vi "GE 5565PIORC.PIO.Endianness.vi"(11 "data type":T1=enum."Single") -> (0 "error out":errorcluster, 3 "pass?":bool)   [LabVIEW 2017]
uses:
  Typedefs/GE 5565PIORC.Data Types.ctl
  Source/GE 5565PIORC.lvclass/GE 5565PIORC.ctl
  Source/Methods/GE 5565PIORC.PIO.Write (SGL).vi
  Source/Methods/GE 5565PIORC.PIO.Read (SGL).vi
  Source/Methods/GE 5565PIORC.PIO.Write (DBL).vi
  Source/Methods/GE 5565PIORC.PIO.Read (DBL).vi
  Source/Methods/GE 5565PIORC.PIO.Write (I16).vi
  Source/Methods/GE 5565PIORC.PIO.Read (I16).vi
  Source/Methods/GE 5565PIORC.PIO.Write (I32).vi
  Source/Methods/GE 5565PIORC.PIO.Read (I32).vi
  Source/Methods/GE 5565PIORC.PIO.Write (I64).vi
  Source/Methods/GE 5565PIORC.PIO.Read (I64).vi
  Source/Methods/GE 5565PIORC.PIO.Write (U16).vi
  Source/Methods/GE 5565PIORC.PIO.Read (U16).vi
  Source/Methods/GE 5565PIORC.PIO.Write (U32).vi
  Source/Methods/GE 5565PIORC.PIO.Read (U32).vi
  Source/Methods/GE 5565PIORC.PIO.Write (U64).vi
  Source/Methods/GE 5565PIORC.PIO.Read (U64).vi
  Source/Methods/GE 5565PIORC.VISA.Move Out.vi
  Source/Methods/GE 5565PIORC.VISA.Move Out.String (U8).vi
  Source/Methods/GE 5565PIORC.VISA.Move In.vi
  Source/Methods/GE 5565PIORC.VISA.Move In.String (U8).vi
  Source/Methods/GE 5565PIORC.VISA.Return Handler.vi
  <vilib>/Utility/error.llb/Error Cluster From Error Code.vi
  Source/GE 5565PIORC.lvclass
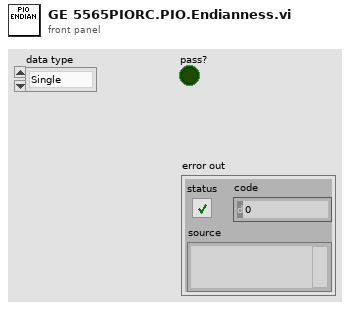
[diagram p1: front panel]
types:
  T1 = typedef "GE 5565PIORC.Data Types.ctl" = enum16{"Boolean", "Single", "Double", "I8", "I16", "I32", "I64", "U8", "U16", "U32", "U64"}
  T2 = enum16{"big-endian, network order", "native, host order", "little-endian"}
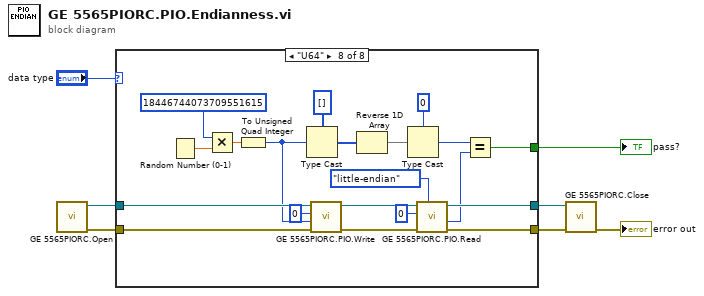
[diagram p0: block diagram]
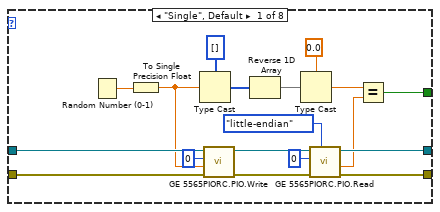
[diagram p2: hidden frame]
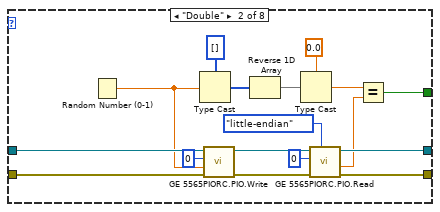
[diagram p3: hidden frame]
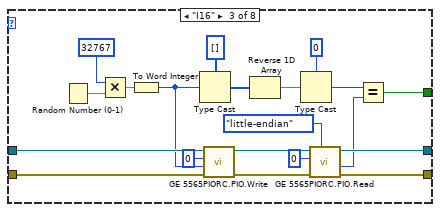
[diagram p4: hidden frame]
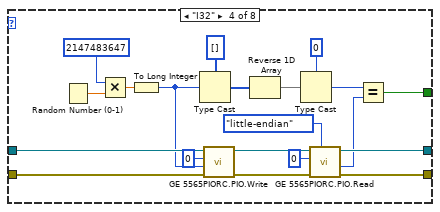
[diagram p5: hidden frame]
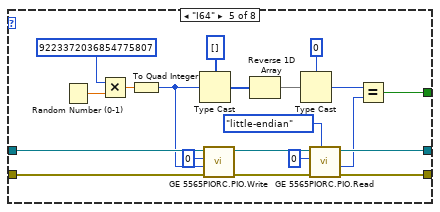
[diagram p6: hidden frame]
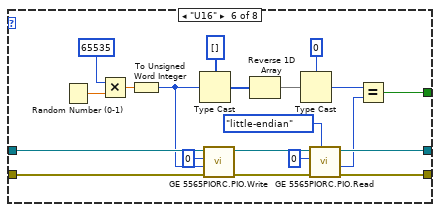
[diagram p7: hidden frame]
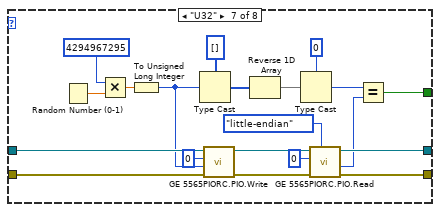
[diagram p8: hidden frame]
diagram:
  n1 = call "GE 5565PIORC.Open.vi"() -> ("error out"=w6:errorcluster, "GE 5565PIORC"=w5:refnum<class "GE 5565PIORC.lvclass">)  [unwired: 10 in]
  n2 = case shown="\"U64\"" "data type" {
    tunnel: w5 -> [w25 w42 w62 w82 w102 w122 w142 w162]
    tunnel: w6 -> [w24 w41 w61 w81 w101 w121 w141 w161]
    tunnel: [w21 w38 w58 w78 w98 w118 w138 w158] -> w4
    tunnel: [w20 w37 w57 w77 w97 w117 w137 w157] -> w3
    tunnel: [w10 w29 w48 w68 w88 w108 w128 w148] -> w1
    frame "Single", Default {
      n3 = Random Number (0-1)() -> (number: 0 to 1=w18:dbl)
      n4 = To Single Precision Float(number=w18) -> (single precision float=w17:sgl)
      n5 = Type Cast(type=u8[] [], x=w17) -> (*(type *) &x=w16:u8[])
      n6 = call-poly "GE 5565PIORC.PIO.Write.vi"("error in (no error)"=w24, "data"=w17, "offset"=u32 0, "GE 5565PIORC in"=w25) -> ("error out"=w22:errorcluster, "GE 5565PIORC out"=w23:refnum<class "GE 5565PIORC.lvclass">)  [unwired: 5 in, 1 out]
      n7 = Reverse 1D Array(array=w16) -> (reversed array=w15:u8[])
      n8 = Type Cast(type=sgl 0.0, x=w15) -> (*(type *) &x=w12:sgl)
      n9 = call-poly "GE 5565PIORC.PIO.Read.vi"("byte order (big-endian)"=T2."little-endian", "error in (no error)"=w22, "offset"=u32 0, "GE 5565PIORC in"=w23) -> ("error out"=w20:errorcluster, "data"=w11:sgl, "GE 5565PIORC out"=w21:refnum<class "GE 5565PIORC.lvclass">)  [unwired: 5 in]
      n10 = Equal?(x=w12, y=w11) -> (x = y?=w10:bool)
    }
    frame "Double" {
      n11 = Random Number (0-1)() -> (number: 0 to 1=w28:dbl)
      n12 = Type Cast(type=u8[] [], x=w28) -> (*(type *) &x=w35:u8[])
      n13 = call-poly "GE 5565PIORC.PIO.Write.vi"("error in (no error)"=w41, "data"=w28, "offset"=u32 0, "GE 5565PIORC in"=w42) -> ("error out"=w39:errorcluster, "GE 5565PIORC out"=w40:refnum<class "GE 5565PIORC.lvclass">)  [unwired: 5 in, 1 out]
      n14 = Reverse 1D Array(array=w35) -> (reversed array=w34:u8[])
      n15 = Type Cast(type=0.0, x=w34) -> (*(type *) &x=w31:dbl)
      n16 = call-poly "GE 5565PIORC.PIO.Read.vi"("byte order (big-endian)"=T2."little-endian", "error in (no error)"=w39, "offset"=u32 0, "GE 5565PIORC in"=w40) -> ("error out"=w37:errorcluster, "data"=w30:dbl, "GE 5565PIORC out"=w38:refnum<class "GE 5565PIORC.lvclass">)  [unwired: 5 in]
      n17 = Equal?(x=w31, y=w30) -> (x = y?=w29:bool)
    }
    frame "I16" {
      n18 = Random Number (0-1)() -> (number: 0 to 1=w46:dbl)
      n19 = Multiply(x=i16 32767, y=w46) -> (x*y=w47:dbl)
      n20 = To Word Integer(number=w47) -> (16bit integer=w55:i16)
      n21 = Type Cast(type=u8[] [], x=w55) -> (*(type *) &x=w54:u8[])
      n22 = call-poly "GE 5565PIORC.PIO.Write.vi"("error in (no error)"=w61, "data"=w55, "offset"=u32 0, "GE 5565PIORC in"=w62) -> ("error out"=w59:errorcluster, "GE 5565PIORC out"=w60:refnum<class "GE 5565PIORC.lvclass">)  [unwired: 5 in, 1 out]
      n23 = Reverse 1D Array(array=w54) -> (reversed array=w53:u8[])
      n24 = Type Cast(type=i16 0, x=w53) -> (*(type *) &x=w50:i16)
      n25 = call-poly "GE 5565PIORC.PIO.Read.vi"("byte order (big-endian)"=T2."little-endian", "error in (no error)"=w59, "offset"=u32 0, "GE 5565PIORC in"=w60) -> ("error out"=w57:errorcluster, "data"=w49:i16, "GE 5565PIORC out"=w58:refnum<class "GE 5565PIORC.lvclass">)  [unwired: 5 in]
      n26 = Equal?(x=w50, y=w49) -> (x = y?=w48:bool)
    }
    frame "I32" {
      n27 = Random Number (0-1)() -> (number: 0 to 1=w66:dbl)
      n28 = Multiply(x=2147483647, y=w66) -> (x*y=w67:dbl)
      n29 = To Long Integer(number=w67) -> (32bit integer=w75:i32)
      n30 = Type Cast(type=u8[] [], x=w75) -> (*(type *) &x=w74:u8[])
      n31 = call-poly "GE 5565PIORC.PIO.Write.vi"("error in (no error)"=w81, "data"=w75, "offset"=u32 0, "GE 5565PIORC in"=w82) -> ("error out"=w79:errorcluster, "GE 5565PIORC out"=w80:refnum<class "GE 5565PIORC.lvclass">)  [unwired: 5 in, 1 out]
      n32 = Reverse 1D Array(array=w74) -> (reversed array=w73:u8[])
      n33 = Type Cast(type=0, x=w73) -> (*(type *) &x=w70:i32)
      n34 = call-poly "GE 5565PIORC.PIO.Read.vi"("byte order (big-endian)"=T2."little-endian", "error in (no error)"=w79, "offset"=u32 0, "GE 5565PIORC in"=w80) -> ("error out"=w77:errorcluster, "data"=w69:i32, "GE 5565PIORC out"=w78:refnum<class "GE 5565PIORC.lvclass">)  [unwired: 5 in]
      n35 = Equal?(x=w70, y=w69) -> (x = y?=w68:bool)
    }
    frame "I64" {
      n36 = Random Number (0-1)() -> (number: 0 to 1=w86:dbl)
      n37 = Multiply(x=i64 9223372036854775807, y=w86) -> (x*y=w87:dbl)
      n38 = To Quad Integer(1:w87) -> (0:w95:i64)
      n39 = Type Cast(type=u8[] [], x=w95) -> (*(type *) &x=w94:u8[])
      n40 = call-poly "GE 5565PIORC.PIO.Write.vi"("error in (no error)"=w101, "data"=w95, "offset"=u32 0, "GE 5565PIORC in"=w102) -> ("error out"=w99:errorcluster, "GE 5565PIORC out"=w100:refnum<class "GE 5565PIORC.lvclass">)  [unwired: 5 in, 1 out]
      n41 = Reverse 1D Array(array=w94) -> (reversed array=w93:u8[])
      n42 = Type Cast(type=i64 0, x=w93) -> (*(type *) &x=w90:i64)
      n43 = call-poly "GE 5565PIORC.PIO.Read.vi"("byte order (big-endian)"=T2."little-endian", "error in (no error)"=w99, "offset"=u32 0, "GE 5565PIORC in"=w100) -> ("error out"=w97:errorcluster, "data"=w89:i64, "GE 5565PIORC out"=w98:refnum<class "GE 5565PIORC.lvclass">)  [unwired: 5 in]
      n44 = Equal?(x=w90, y=w89) -> (x = y?=w88:bool)
    }
    frame "U16" {
      n45 = Random Number (0-1)() -> (number: 0 to 1=w106:dbl)
      n46 = Multiply(x=u16 65535, y=w106) -> (x*y=w107:dbl)
      n47 = To Unsigned Word Integer(number=w107) -> (unsigned 16bit integer=w115:u16)
      n48 = Type Cast(type=u8[] [], x=w115) -> (*(type *) &x=w114:u8[])
      n49 = call-poly "GE 5565PIORC.PIO.Write.vi"("error in (no error)"=w121, "data"=w115, "offset"=u32 0, "GE 5565PIORC in"=w122) -> ("error out"=w119:errorcluster, "GE 5565PIORC out"=w120:refnum<class "GE 5565PIORC.lvclass">)  [unwired: 5 in, 1 out]
      n50 = Reverse 1D Array(array=w114) -> (reversed array=w113:u8[])
      n51 = Type Cast(type=u16 0, x=w113) -> (*(type *) &x=w110:u16)
      n52 = call-poly "GE 5565PIORC.PIO.Read.vi"("byte order (big-endian)"=T2."little-endian", "error in (no error)"=w119, "offset"=u32 0, "GE 5565PIORC in"=w120) -> ("error out"=w117:errorcluster, "data"=w109:u16, "GE 5565PIORC out"=w118:refnum<class "GE 5565PIORC.lvclass">)  [unwired: 5 in]
      n53 = Equal?(x=w110, y=w109) -> (x = y?=w108:bool)
    }
    frame "U32" {
      n54 = Random Number (0-1)() -> (number: 0 to 1=w126:dbl)
      n55 = Multiply(x=u32 4294967295, y=w126) -> (x*y=w127:dbl)
      n56 = To Unsigned Long Integer(number=w127) -> (unsigned 32bit integer=w135:u32)
      n57 = Type Cast(type=u8[] [], x=w135) -> (*(type *) &x=w134:u8[])
      n58 = call-poly "GE 5565PIORC.PIO.Write.vi"("error in (no error)"=w141, "data"=w135, "offset"=u32 0, "GE 5565PIORC in"=w142) -> ("error out"=w139:errorcluster, "GE 5565PIORC out"=w140:refnum<class "GE 5565PIORC.lvclass">)  [unwired: 5 in, 1 out]
      n59 = Reverse 1D Array(array=w134) -> (reversed array=w133:u8[])
      n60 = Type Cast(type=u32 0, x=w133) -> (*(type *) &x=w130:u32)
      n61 = call-poly "GE 5565PIORC.PIO.Read.vi"("byte order (big-endian)"=T2."little-endian", "error in (no error)"=w139, "offset"=u32 0, "GE 5565PIORC in"=w140) -> ("error out"=w137:errorcluster, "data"=w129:u32, "GE 5565PIORC out"=w138:refnum<class "GE 5565PIORC.lvclass">)  [unwired: 5 in]
      n62 = Equal?(x=w130, y=w129) -> (x = y?=w128:bool)
    }
    frame "U64" {
      n63 = Random Number (0-1)() -> (number: 0 to 1=w146:dbl)
      n64 = Multiply(x=u64 18446744073709551615, y=w146) -> (x*y=w147:dbl)
      n65 = To Unsigned Quad Integer(1:w147) -> (0:w155:u64)
      n66 = Type Cast(type=u8[] [], x=w155) -> (*(type *) &x=w154:u8[])
      n67 = call-poly "GE 5565PIORC.PIO.Write.vi"("error in (no error)"=w161, "data"=w155, "offset"=u32 0, "GE 5565PIORC in"=w162) -> ("error out"=w159:errorcluster, "GE 5565PIORC out"=w160:refnum<class "GE 5565PIORC.lvclass">)  [unwired: 5 in, 1 out]
      n68 = Reverse 1D Array(array=w154) -> (reversed array=w153:u8[])
      n69 = Type Cast(type=u64 0, x=w153) -> (*(type *) &x=w150:u64)
      n70 = call-poly "GE 5565PIORC.PIO.Read.vi"("byte order (big-endian)"=T2."little-endian", "error in (no error)"=w159, "offset"=u32 0, "GE 5565PIORC in"=w160) -> ("error out"=w157:errorcluster, "data"=w149:u64, "GE 5565PIORC out"=w158:refnum<class "GE 5565PIORC.lvclass">)  [unwired: 5 in]
      n71 = Equal?(x=w150, y=w149) -> (x = y?=w148:bool)
    }
  }
  "pass?" <- w1
  n72 = call "GE 5565PIORC.Close.vi"("error in (no error)"=w3, "GE 5565PIORC"=w4) -> ("error out"=→"error out":errorcluster)  [unwired: 9 in]
